vi "Generate Command String.vi"(8 "error in (no error)":errorcluster, 10 "Value":u16, 11 "Command":u16) -> (0 "error out":errorcluster, 3 "Command String":string)   [LabVIEW 2013]
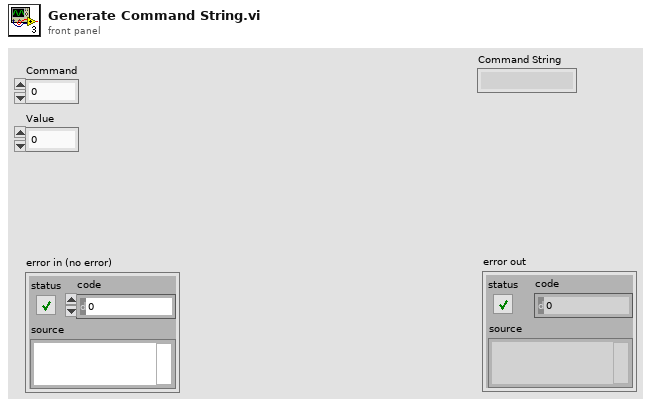
[diagram p1: front panel]
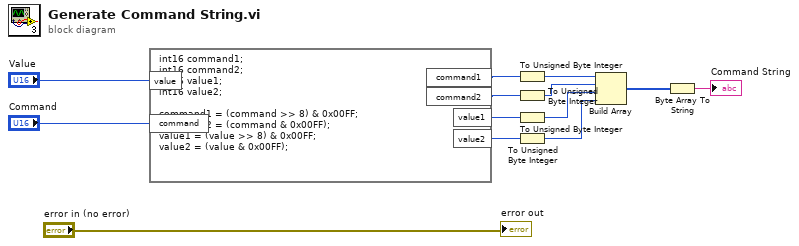
[diagram p0: block diagram]
diagram:
  n1 = formula code="int16 command1;\nint16 command2;\nint16 value1;\nint16 value2;\n\ncommand1 = (command >> 8) & 0x00FF;\ncommand2 = (command & 0x00FF);\nvalue1 = (value >> 8) & 0x00FF;\nvalue2 = (value & 0x00FF);"("command"="Command", "value"="Value") -> ("command1"=w12:i16, "command2"=w11:i16, "value1"=w10:i16, "value2"=w9:i16)
  n2 = To Unsigned Byte Integer(number=w12) -> (unsigned 8bit integer=w13:u8)
  n3 = To Unsigned Byte Integer(number=w11) -> (unsigned 8bit integer=w8:u8)
  n4 = To Unsigned Byte Integer(number=w10) -> (unsigned 8bit integer=w7:u8)
  n5 = To Unsigned Byte Integer(number=w9) -> (unsigned 8bit integer=w6:u8)
  n6 = Build Array(w13, w8, w7, w6) -> (w5:u8[])
  n7 = Byte Array To String(unsigned byte array=w5) -> (string=→"Command String":string)
  "error out" <- "error in (no error)"
